vi "PD Offset.vi"() -> ()   [LabVIEW 2018]
uses:
  <vilib>/Analysis/baseanly.llb/Mean (DBL).vi
  <vilib>/Analysis/NI_AALBase.lvlib
panel:
  in  "number of samples":i32=5000
  in  "Filename":path=path "C:/Users/physics-svc-fulda/Desktop/LabVIEW Data/PD OFFset.lvm"
  out "data":dynamicdata(graph)
  out "PD Offset":dbl format="%0.6f"
  out "Saving Data":bool
  in  "Enable":bool=TRUE
  in  "timeout (s)":dbl=10.0 format="%0.2f"
  in  "rate":dbl=1000.0
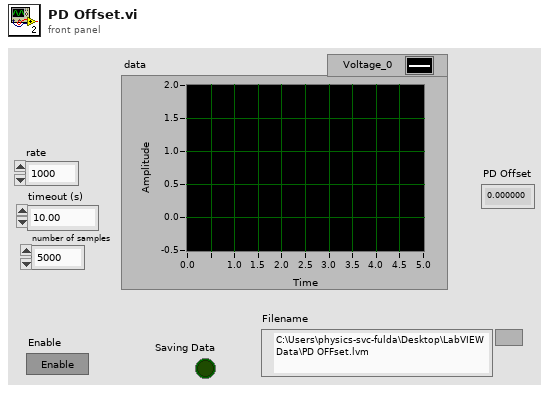
[diagram p1: front panel]
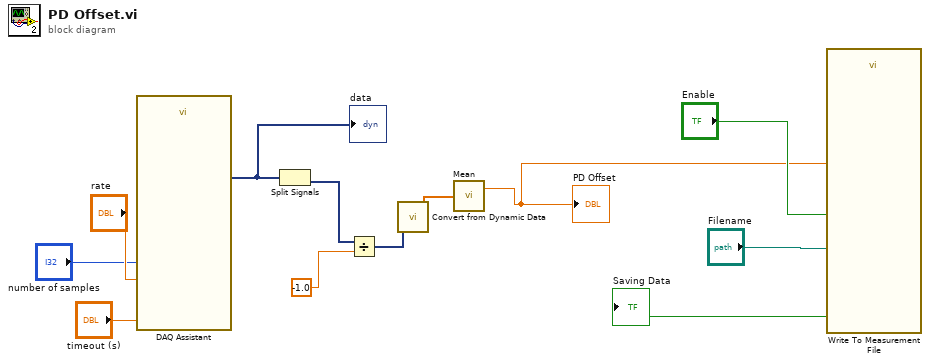
[diagram p0: block diagram]
diagram:
  n1 = call "DAQ Assistant"("rate"="rate", "number of samples"="number of samples", "timeout (s)"="timeout (s)") -> ("data"=w10:dynamicdata)  [unwired: 14 in, 2 out]
  "data" <- w10
  n2 = Split Signals(w10) -> (w4:dynamicdata)  [unwired: 2 in, 1 out]
  n3 = Divide(x=w4, y=-1.0) -> (x/y=w3:dynamicdata)
  n4 = call "Convert from Dynamic Data"("Dynamic Data Type"=w3) -> ("Array"=w7:dbl[])  [unwired: 3 in]
  n5 = call-poly <vilib>:"Mean.vi"("X"=w7) -> ("mean"=w6:dbl)  [unwired: 1 out]
  "PD Offset" <- w6
  n6 = call "Write To Measurement File"("Signals"=w6, "Enable"="Enable", "Filename"="Filename") -> ("Saving Data"=→"Saving Data":bool)  [unwired: 14 in, 2 out]
